vi "StepDefault.vi"(7 "Action":string, 11 "error in":errorcluster) -> (8 "Results":T1, 15 "error out":errorcluster)   [LabVIEW 2021]
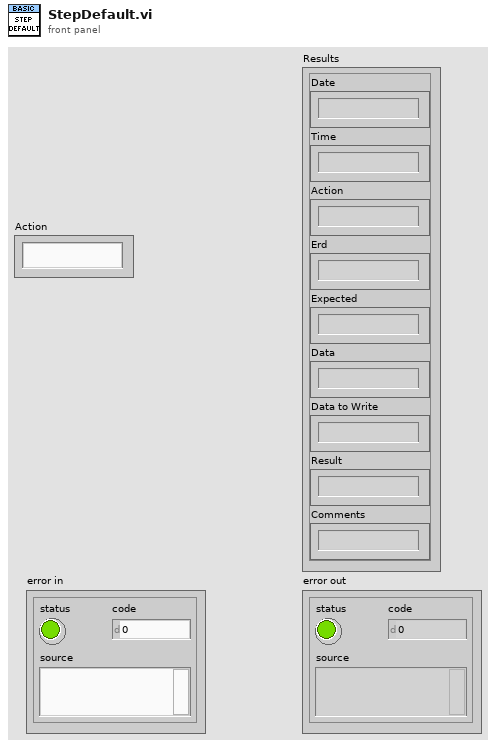
[diagram p1: front panel]
types:
  T1 = cluster{"Date":string, "Time":string, "Action":string, "Erd":string, "Expected":string, "Data":string, "Data to Write":string, "Result":string, "Comments":string}
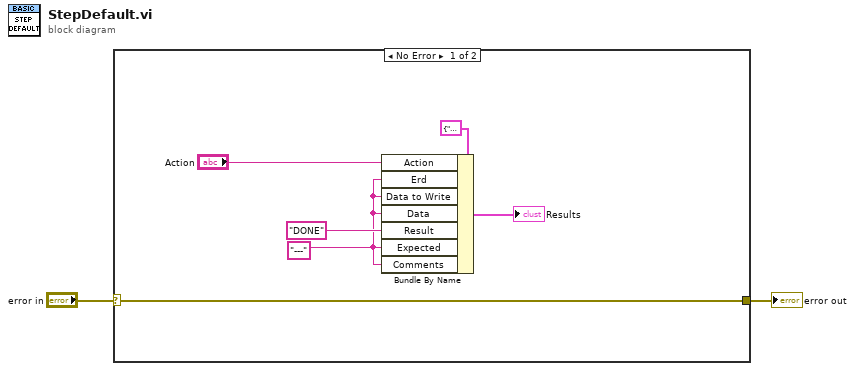
[diagram p0: block diagram]
diagram:
  n1 = case shown="No Error" "error in" {
    selector: "error in" -> [w5 w9]
    tunnel: [w5 w9] -> w1
    frame No Error {
      w3 = "---"
      n2 = Bundle By Name(cluster=T1 {"Date"="", "Time"="", "Action"="", "Erd"="", "Expected"="", "Data"="", "Data to Write"="", "Result"="", "Comments"=""}, "Action"="Action", "Erd"=w3, "Data to Write"=w3, "Data"=w3, "Result"="DONE", "Expected"=w3, "Comments"=w3) -> (→"Results":T1)
    }
    frame Error {
    }
  }
  "error out" <- w1
